vi "Query Sweep Points.vi"(8 "error in (no error)":errorcluster, 11 "VISA resource name":refnum<visa-resource-name>) -> (0 "error out":errorcluster, 2 "Number of Sweep Points":i32, 3 "VISA resource name out":refnum<visa-resource-name>)   [LabVIEW 2012, in "Agilent PSG MXG Series.lvlib"]
uses:
  Agilent PSG MXG Series.lvlib
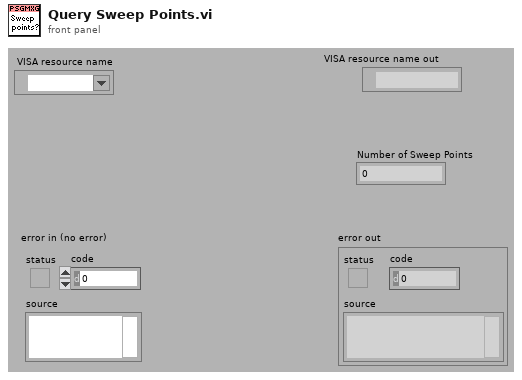
[diagram p1: front panel]
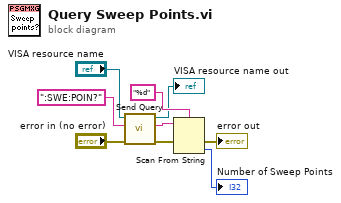
[diagram p0: block diagram]
diagram:
  n1 = call "Send Query.vi"("error in (no error)"="error in (no error)", "write buffer"=":SWE:POIN?", "VISA resource name"="VISA resource name") -> ("error out"=w2:errorcluster, "read buffer"=w6:string, "VISA resource name out"=→"VISA resource name out":refnum<visa-resource-name>)  [unwired: 6 out]
  n2 = Scan From String(format string="%d", input string=w6, error in=w2) -> (error out=→"error out":errorcluster, output 1=→"Number of Sweep Points":i32)  [unwired: 1 in, 3 out]
